vi "Digital Read Pin.vi"(0 "Arduino Resource":T1={"VISA resource"="", "Board Type"=enum."Uno", "Connection Type"=enum."USB / Serial", "Bytes Per Packet (15)"=15}, 7 "Digital I/O Pin (0)":u8, 11 "error in":errorcluster) -> (4 "Arduino Resource":T1={"VISA resource"="", "Board Type"=enum."Uno", "Connection Type"=enum."USB / Serial", "Bytes Per Packet (15)"=15}, 8 "Value":u8, 15 "error out":errorcluster)   [LabVIEW 2011, in "LabVIEW Interface for Arduino.lvlib"]
doc: "Reads the digital value of the selected Arduino digital input pin (D0 - D13). The pin must fist be configured as an input using the Arduino Set Digital Pin Mode VI."
uses:
  <vilib>/LabVIEW Interface for Arduino/LabVIEW Interface for Arduino.lvlib
  <vilib>/LabVIEW Interface for Arduino/Private/Type Defs/Arduino Resource.ctl
  <vilib>/LabVIEW Interface for Arduino/Private/Type Defs/Board Type.ctl
  <vilib>/LabVIEW Interface for Arduino/Private/Type Defs/Command.ctl
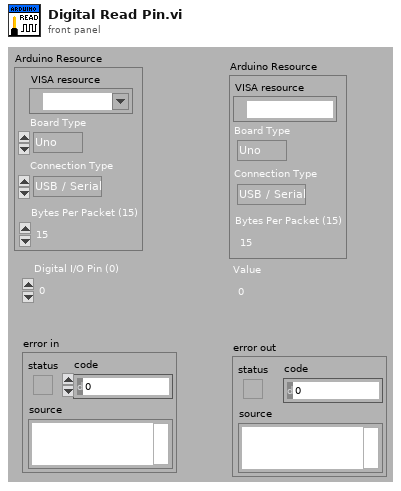
[diagram p1: front panel]
types:
  T1 = typedef "LabVIEW Interface for Arduino.lvlib/Arduino Resource.ctl" = cluster{"VISA resource":refnum<visa-resource-name>, "Board Type":T2, "Connection Type":enum8{"USB / Serial"}, "Bytes Per Packet (15)":u8}
  T2 = typedef "LabVIEW Interface for Arduino.lvlib/Board Type.ctl" = enum16{"Uno", "Dimuelanove w/Atmega 328", "Mega 2560"}
  T3 = typedef "LabVIEW Interface for Arduino.lvlib/Command.ctl" = enum8{"setArduinoMode", "flushSerial", "setPinMode", "digitalWritePin", "digitalWritePort", "tone", "digitalReadPin", "digitalReadPort", "analogReadPin", "analogReadPort", "pwmWritePin", "pwmWritePort", "sevenSegment_Configure", "sevenSegment_Write", "I2C Init", "I2C Write", "I2C Read", "SPI Init", "SPI Set Bit Order", "SPI Set Clock Divider", "SPI Set Data Mode", "SPI Send / Receive", "SPI Close", "Servo Set Num Servos", "Servo Config Servo", "Servo Write Angle", "Servo Read Angle", "Servo Write Pulse Width", "Servo Read Pulse Width", "Servo Detach", "LCD Init", "LCD Set Size", "LCD Set Cursor Mode", "LCD Clear", "LCD Set Cursor Position", "LCD Print", "LCD Display Power", "LCD Scroll Display", "LCD Autoscroll", "LCD Print Direction", "LCD Create Custom Char", "LCD Print Custom Char", "contAcqOn", "contAcqOff", "getFirmwareVersion", "FiniteSampleStart"}
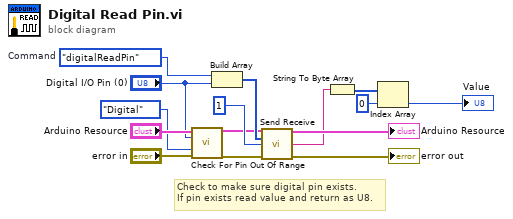
[diagram p0: block diagram]
diagram:
  w15 = Command."digitalReadPin"  # Command
  # "Check to make sure digital pin exists.\nIf pin exists read value and return as U8."
  n1 = call <vilib>:"Check For Pin Out Of Range.vi"("Arduino Resource"="Arduino Resource", "User Pin Number"="Digital I/O Pin (0)", "Pin Type"=enum16{"Analog", "Digital"}."Digital", "error in"="error in") -> ("Arduino Resource"=w9:T1, "error out"=w8:errorcluster)  [unwired: 10 in]
  n2 = Build Array(w15, "Digital I/O Pin (0)") -> (w12:u8[])
  n3 = call <vilib>:"Send Receive.vi"("Arduino Resource"=w9, "Data"=w12, "Bytes To Read (0)"=u32 1, "error in"=w8) -> ("Arduino Resource"=→"Arduino Resource":T1, "Read Buffer"=w4:string, "error out"=→"error out":errorcluster)  [unwired: 9 in]
  n4 = String To Byte Array(string=w4) -> (unsigned byte array=w3:u8[])
  n5 = Index Array(array=w3, index=0) -> (element=→"Value":u8)
